vi "Initialize.vi"(7 "fluidics line":string="Dev1/port2/line6", 8 "error in (no error)":errorcluster, 9 "Shutter Lines":string[](array[string]), 10 "Sync Line":string, 11 "Synchronization Device in":refnum<class "Sync Device.lvclass">) -> (0 "error out":errorcluster, 3 "Synchronization Device out":refnum<class "Sync Device.lvclass">)   [LabVIEW 2023, in "Sync Device.lvlib" / "Sync Device.lvclass"]
uses:
  Sync Device.lvclass
  Sync Device.lvclass/Sync Device.ctl
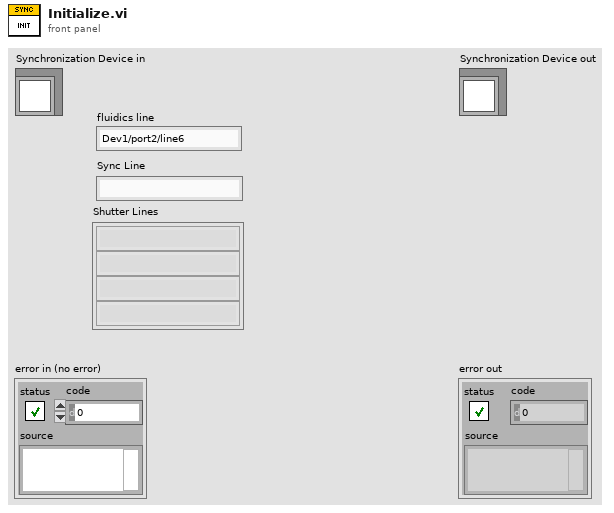
[diagram p1: front panel]
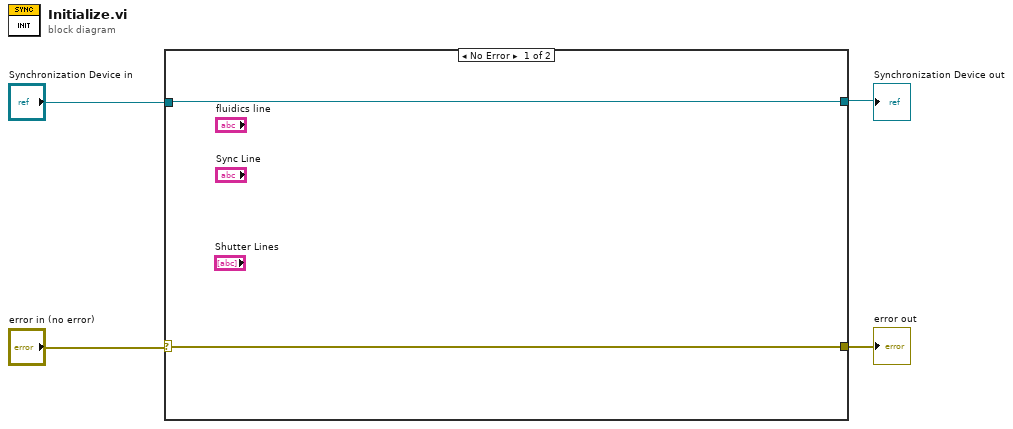
[diagram p0: block diagram]
diagram:
  n1 = case shown="No Error" "error in (no error)" {
    selector: "error in (no error)" -> [w6 w8]
    tunnel: [w6 w8] -> w3
    tunnel: [w5 w7] -> w1
    tunnel: "Synchronization Device in" -> [w5 w7]
    frame No Error {
    }
    frame Error {
    }
  }
  "error out" <- w3
  "Synchronization Device out" <- w1
